vi "FindHome.vi"(0 "Axis In":T1, 5 "Type":T2(ring), 11 "error in (no error)":errorcluster) -> (4 "Axis Out":T1, 15 "error out":errorcluster)   [LabVIEW 2009]
uses:
  typedefs/Ultra3000/Func.ctl
  typedefs/Ultra3000/Cmds.ctl
  typedefs/AxisSelect_Enum.ctl
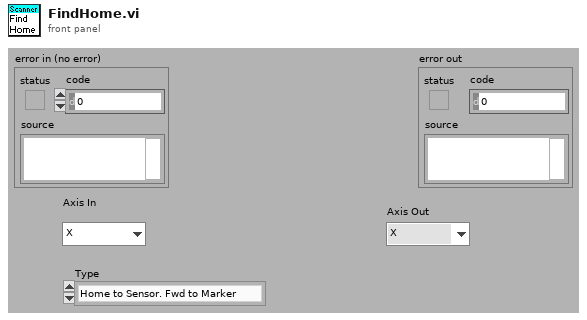
[diagram p1: front panel]
types:
  T1 = typedef "AxisSelect_Enum.ctl" = enum16{"X", "Y", "Z", "Axis Space"}
  T2 = enum16{"Home to Sensor. Fwd to Marker", "Home to Marker", "Home to Sensor", "Home to sensor, backward to maker", "Home to current setting", "Home to current setting, backward to marker"}
  T3 = typedef "Func.ctl" = u16
  T4 = typedef "Cmds.ctl" = u16
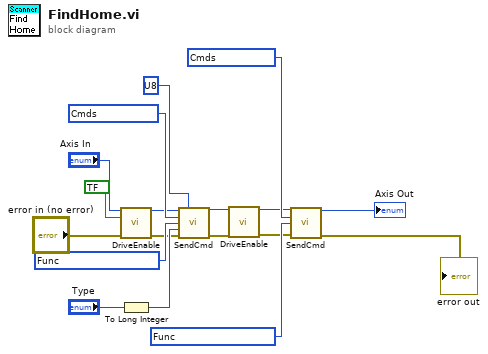
[diagram p0: block diagram]
diagram:
  w8 = T3 ? items=["Read Working Value", "Write Working Value", "Read Non-Volatile Value", "Write Non-Volatile and Woring Value", "Copy Non-Volatile Value to Working Value", "Copy Working Value to Non-Volatile Value", "Read Default Value", "Copy Default Value to Non-Volatile and Working Values", "Read Min Value", "Read Max Value", "Read Array Index Min", "Read Array Index Max"] ("Function")
  w9 = T4 ? items=["Drive Status", "Position Command", "Run Status", "Fault Status", "Position Error", "Auto-Start Homing", "Start Homing", "Homing Type", "Motor Position", "Velocity Motor", "Power-Up Status", "Drive Name", "Position Window Size", "Position Window Time", "Zero Speed Limit", "Speed Window Size", "Up to Speed Limit", "Forward Current Limit", "Reverse Current Limit", "Override Mode", "Operation Mode", "Host Control Mode", "Reset Drive", "Drive Enable", "Setpoint Current", "Setpoint Velocity", "Setpoint Acceleration", "Reset Faults", "Position Comparator", "Postition Comparator Polarity", "Position Rollover Enable", "Baud Rate", "Frame Format", "Drive Address", "Broadcast Address", "Auto-start Indexing", "Start Index", "Host Index", "Index Type", "Index Dist/Pos", "Index Reg Dist", "Index Velocity", "Index Acceleration", "Index Deceleration", "Index Dwell", "Index Count", "Index Termination", "Index Pointer", "Index Abort Deceleration", "Positive Soft Pos Limit", "Define Home", "Negative Soft Pos Limit"] ("Command")
  w12 = T4 ? items=["Start Homing", "Homing Type", "Motor Position", "Velocity Motor", "Power-Up Status", "Drive Name", "Position Window Size", "Position Window Time", "Zero Speed Limit", "Speed Window Size", "Up to Speed Limit", "Forward Current Limit", "Reverse Current Limit", "Override Mode", "Operation Mode", "Host Control Mode", "Reset Drive", "Drive Enable", "Setpoint Current", "Setpoint Velocity", "Setpoint Acceleration", "Reset Faults", "Position Comparator", "Postition Comparator Polarity", "Position Rollover Enable", "Baud Rate", "Frame Format", "Drive Address", "Broadcast Address", "Auto-start Indexing", "Start Index", "Host Index", "Index Type", "Index Dist/Pos", "Index Reg Dist", "Index Velocity", "Index Acceleration", "Index Deceleration", "Index Dwell", "Index Count", "Index Termination", "Index Pointer", "Index Abort Deceleration", "Positive Soft Pos Limit", "Define Home", "Negative Soft Pos Limit"] ("Command")
  w16 = T3 ? items=["Read Working Value", "Write Working Value", "Read Non-Volatile Value", "Write Non-Volatile and Woring Value", "Copy Non-Volatile Value to Working Value", "Copy Working Value to Non-Volatile Value", "Read Default Value", "Copy Default Value to Non-Volatile and Working Values", "Read Min Value", "Read Max Value", "Read Array Index Min", "Read Array Index Max"] ("Function")
  n1 = call "DriveEnable.vi"("Axis In (Axis Space)"="Axis In", "Enable (T)"=bool ? ("Boolean"), "error in (no error)"="error in (no error)") -> ("Axis Out"=w11:T1, "error out"=w10:errorcluster)  [unwired: 11 in]
  n2 = To Long Integer(number="Type") -> (32bit integer=w13:i32)
  n3 = call "SendCmd.vi"("Axis In"=w11, "Data Length Constant (0)"=u8 ? ("DLC"), "Command"=w12, "Function"=w16, "Data (0)"=w13, "error in (no error)"=w10) -> ("Axis Out"=w7:T1, "error out"=w6:errorcluster)  [unwired: 6 in, 2 out]
  n4 = call "DriveEnable.vi"("Axis In (Axis Space)"=w7, "error in (no error)"=w6) -> ("Axis Out"=w4:T1, "error out"=w5:errorcluster)  [unwired: 12 in]
  n5 = call "SendCmd.vi"("Axis In"=w4, "Command"=w9, "Function"=w8, "error in (no error)"=w5) -> ("Axis Out"=→"Axis Out":T1, "error out"=→"error out":errorcluster)  [unwired: 8 in, 2 out]
